vi "Write modbus type.vi"(8 "error in":errorcluster, 10 "modbus type":T1, 11 "Modbus Module Channel in":refnum<class "Modbus Module Channel.lvclass">) -> (0 "error out":errorcluster, 3 "Modbus Module Channel out":refnum<class "Modbus Module Channel.lvclass">)   [LabVIEW 2013, in "Modbus Module Channel.lvclass"]
uses:
  Modbus Module Channel.lvclass
  data bank type.ctl
  Modbus Module Channel.lvclass/Modbus Module Channel.ctl
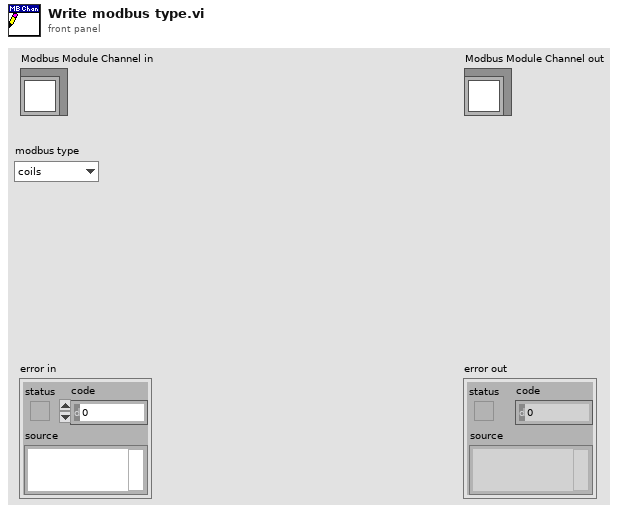
[diagram p1: front panel]
types:
  T1 = typedef "Modbus Module Channel.lvclass/data bank type.ctl" = enum16{"coils", "discrete inputs", "input registers", "holding registers"}
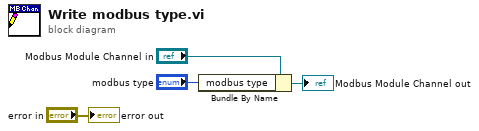
[diagram p0: block diagram]
diagram:
  n1 = Bundle By Name(cluster="Modbus Module Channel in", "modbus type"="modbus type") -> (→"Modbus Module Channel out":refnum<class "Modbus Module Channel.lvclass">)
  "error out" <- "error in"
